vi "Core Action.vi"(8 "error in (no error)":errorcluster, 10 "SECS-II Class":refnum<class "SECS-II Class.lvclass">, 11 "20-Process Program Downloading in":refnum<class "20-Process Program Downloading.lvclass">) -> (0 "error out":errorcluster, 2 "SECS-II Class Out":refnum<class "SECS-II Class.lvclass">, 3 "20-Process Program Downloading out":refnum<class "20-Process Program Downloading.lvclass">)   [LabVIEW 2020, in "SECS Scenarios.lvlib" / "20-Process Program Downloading.lvclass"]
uses:
  20-Process Program Downloading.lvclass
  D:/Dropbox/SECS/SECS_GEM v1.1.0/Com/SECS Scenarios/Scenarios Class/Scenarios Class.lvclass
  SECS Communication/SECS-II Class/SECS-II Class.lvclass
  Scenarios Class/Reply State.ctl
  Scenarios Class/Scenarios Class.lvclass/Scenarios Class.ctl
  Scenarios Class/Write Reply State.vi
  Scenarios Class/Scenarios Class.lvclass
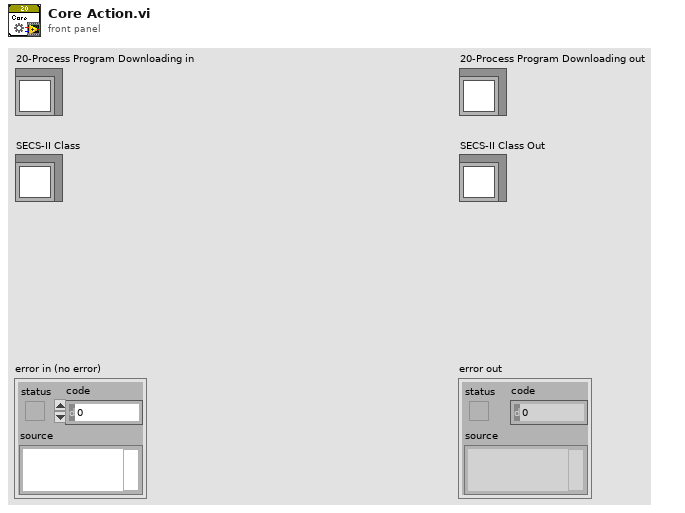
[diagram p1: front panel]
types:
  T1 = typedef "SECS Scenarios.lvlib/Scenarios Class.lvclass/Reply State.ctl" = enum16{"OK", "Illegal Data", "Unknown Stream", "Unknown Function", "Off-Line", "T3 Timeout", "Inner-Timeout"}
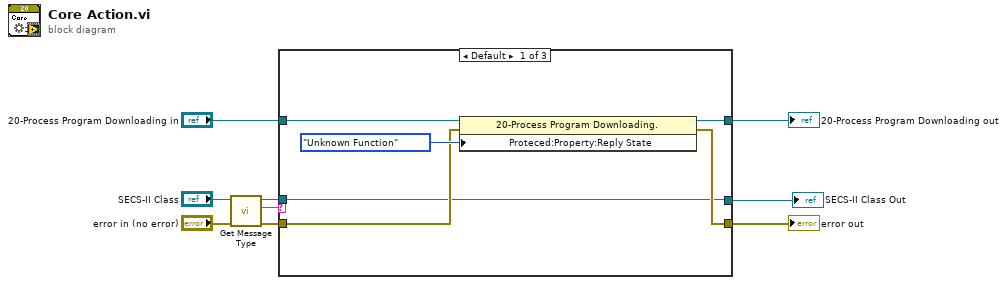
[diagram p0: block diagram]
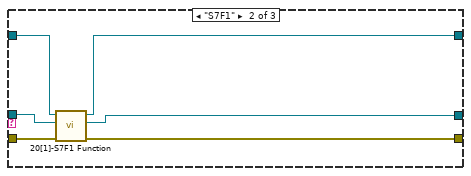
[diagram p2: hidden frame]
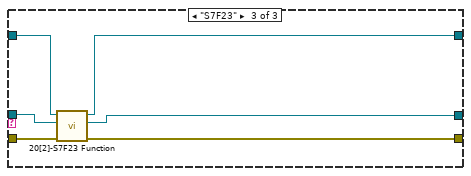
[diagram p3: hidden frame]
diagram:
  n1 = call "Get Message Type.vi"("error in (no error)"="error in (no error)", "SECS-II Class in"="SECS-II Class") -> ("error out"=w6:errorcluster, "Message Type"=w7:string, "SECS-II Class out"=w5:refnum<class "SECS-II Class.lvclass">)  [unwired: 6 in, 1 out]
  n2 = case shown="Default" w7 {
    tunnel: w6 -> [w11 w21 w27]
    tunnel: w5 -> [w10 w20 w26]
    tunnel: "20-Process Program Downloading in" -> [w15 w19 w25]
    tunnel: [w13 w18 w24] -> w3
    tunnel: [w12 w17 w23] -> w2
    tunnel: [w10 w16 w22] -> w1
    frame Default {
      n3 = property class="20-Process Program Downloading."(reference=w15, error in=w11, "Proteced:Property:Reply State"=Reply_State."Unknown Function" ("Reply State")) -> (reference out=w13:refnum<class "20-Process Program Downloading.lvclass">, error out=w12:errorcluster)
    }
    frame "S7F1" {
      n4 = call "20[1]-S7F1 Function.vi"("error in (no error)"=w21, "SECS-II Class"=w20, "20-Process Program Downloading in"=w19) -> ("error out"=w17:errorcluster, "SECS-II Class Out"=w16:refnum<class "SECS-II Class.lvclass">, "20-Process Program Downloading out"=w18:refnum<class "20-Process Program Downloading.lvclass">)  [unwired: 6 in]
    }
    frame "S7F23" {
      n5 = call "20[2]-S7F23 Function.vi"("error in (no error)"=w27, "SECS-II Class"=w26, "20-Process Program Downloading in"=w25) -> ("error out"=w23:errorcluster, "SECS-II Class Out"=w22:refnum<class "SECS-II Class.lvclass">, "20-Process Program Downloading out"=w24:refnum<class "20-Process Program Downloading.lvclass">)  [unwired: 6 in]
    }
  }
  "error out" <- w2
  "20-Process Program Downloading out" <- w3
  "SECS-II Class Out" <- w1
